vi "setColumn.vi"(7 "bus":T1, 8 "error in":errorcluster) -> (0 "error out":errorcluster)   [LabVIEW 2020]
uses:
  bus.ctl
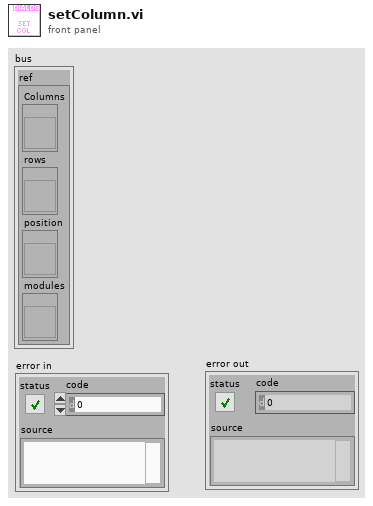
[diagram p1: front panel]
types:
  T1 = typedef "bus.ctl" = cluster{"ref":cluster{"Columns":refnum<vi>, "rows":refnum<vi>, "position":refnum<vi>, "modules":refnum<vi>}}
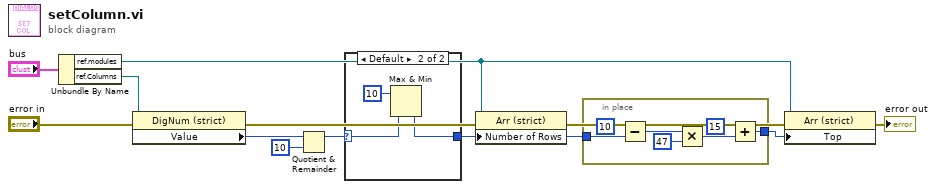
[diagram p0: block diagram]
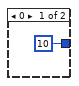
[diagram p2: hidden frame]
diagram:
  n1 = Unbundle By Name("bus") -> ("ref.modules"=w6:refnum<vi>, "ref.Columns"=w9:refnum<vi>)
  n2 = property class="DigNum (strict)"(reference=w9, error in="error in") -> (error out=w12:errorcluster, "Value"=w2:u8)  [unwired: 1 out]
  n3 = Quotient & Remainder(x=w2, y=u8 10) -> (x-y*floor(x/y)=w1:u8)  [unwired: 1 out]
  n4 = case shown="Default" w1 {
    selector: w1 -> [_ w14]
    tunnel: [u8 10 w15] -> w4
    frame 0 {
    }
    frame Default {
      n5 = Max & Min(x=u8 10, y=w14) -> (min(x,y)=w15:u8)  [unwired: 1 out]
    }
  }
  n6 = property on="Property Node" class="Arr (strict)"(reference=w6, error in=w12, "Number of Rows"=w4) -> (error out=w10:errorcluster)  [unwired: 1 out]
  n7 = in-place {
    in-place-border: [w18] -> w5
    in-place-border: w4 -> [w17]
    n8 = Subtract(x=10, y=w17) -> (x-y=w23:i32)
    n9 = Multiply(x=w23, y=47) -> (x*y=w21:i32)
    n10 = Add(x=15, y=w21) -> (x+y=w18:i32)
  }
  n11 = property on="Property Node" class="Arr (strict)"(reference=w6, error in=w10, "Top"=w5) -> (error out=→"error out":errorcluster)  [unwired: 1 out]
